vi "Example_Histogram_HVI.vi"() -> ()   [LabVIEW 2013]
uses:
  Instance           4 29Saved   Example_Histogram_HVI .vi
panel:
  in  "Time Offset":i64
  out "Rate Counter":i32
  in  "Bins":i32=100
  in  "BinSize":i32=9
  in  "Stop Channel":i32=1
  in  "Start Channel":i32
  in  "nHistogram":i32
  out "Close Status":errorcluster
  in  "Stop Loop":bool
  out "histogramVector":i32[](array[numeric])
  out "HistogramPlot":u32[](graph)
  out "HistogramRead Status":errorcluster
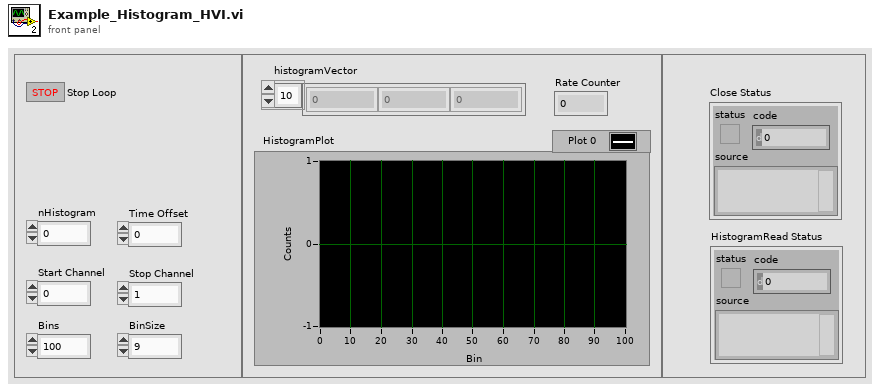
[diagram p1: front panel]
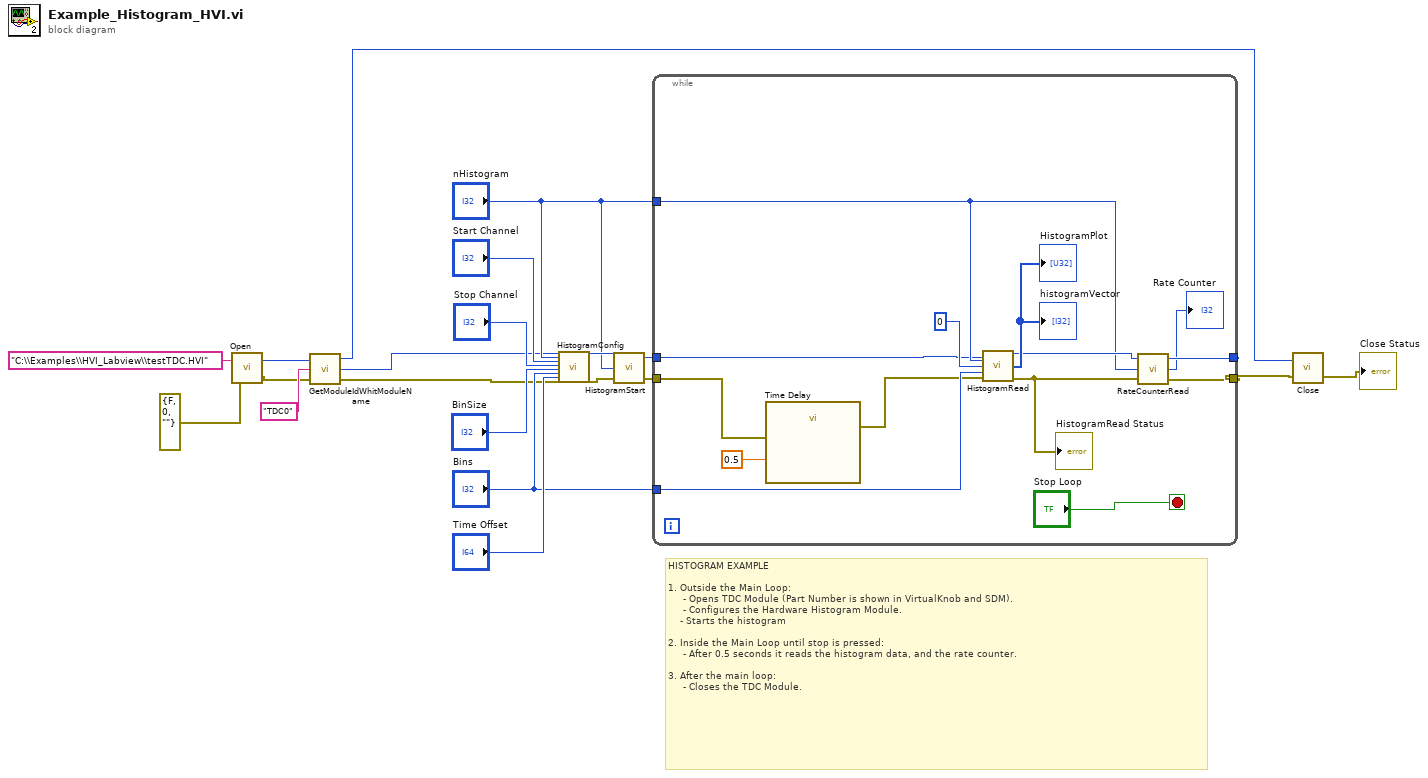
[diagram p0: block diagram]
diagram:
  # "HISTOGRAM EXAMPLE\n\n1. Outside the Main Loop:\n     - Opens TDC Module (Part Number is shown in VirtualKnob and SDM).\n     - Configures the Hardware Histogram Module.\n    - Starts the histogram\n\n2. Inside the Main Loop until stop is pressed:\n     - After 0.5 seconds it reads the histogram data, and the rate counter.\n\n3. After the main loop:\n     - Closes the TDC Module."
  n1 = call <vilib>:"Open.vi"("errorIn"=errorcluster {"status"=FALSE, "code"=0, "source"=""}, "HVIfile"="C:\\Examples\\HVI_Labview\\testTDC.HVI") -> ("errorOut"=w6:errorcluster, "HVIID"=w8:i32)
  n2 = call <vilib>:"GetModuleIdWhitModuleName.vi"("errorIn"=w6, "ModuleName"="TDC0", "HVIID"=w8) -> ("errorOut"=w4:errorcluster, "ModuleID"=w5:u32, "HVIIDOut"=w1:i32)
  n3 = call <vilib>:"HistogramConfig.vi"("moduleID"=w5, "nHistogram"="nHistogram", "startChannel"="Start Channel", "stopChannel"="Stop Channel", "binSize"="BinSize", "nBins"="Bins", "timeOffset"="Time Offset", "errorIn"=w4) -> ("moduleIDout"=w15:i32, "errorOut"=w14:errorcluster)  [unwired: 18 in]
  n4 = call <vilib>:"HistogramStart.vi"("errorIn"=w14, "nHistogram"="nHistogram", "moduleID"=w15) -> ("errorOut"=w13:errorcluster, "moduleIDout"=w12:i32)  [unwired: 1 in]
  n5 = while {
    tunnel: [w29] -> _
    tunnel: [w30] -> w3
    tunnel: "nHistogram" -> [w25]
    tunnel: "Bins" -> [w28]
    tunnel: w13 -> [w22]
    tunnel: w12 -> [w21]
    stop <- "Stop Loop" stop-if-true
    n6 = call "Time Delay"("error in (no error)"=w22, "Delay Time (s)"=0.5) -> ("error out"=w23:errorcluster)  [unwired: 9 in]
    n7 = call <vilib>:"HistogramRead.vi"("moduleID"=w21, "nHistogram"=w25, "startBin"=0, "nBins"=w28, "errorIn"=w23) -> ("moduleIDout"=w27:i32, "histogramData"=→"histogramVector" →"HistogramPlot":u32[], "errorOut"=w26:errorcluster)  [unwired: 8 in]
    "HistogramRead Status" <- w26
    n8 = call <vilib>:"RateCounterRead.vi"("errorIn"=w26, "nChannel"=w25, "moduleID"=w27) -> ("errorOut"=w30:errorcluster, "countRate"=→"Rate Counter":i32, "moduleIDout"=w29:i32)
  }
  n9 = call <vilib>:"Close.vi"("errorIn"=w3, "moduleID"=w1) -> ("errorOut"=→"Close Status":errorcluster)  [unwired: 1 in]
